vi "Random choice.vi"(11 "Selection Made":bool) -> (0 "Number Choice":dbl, 1 "shuffled names":string[](array[string]), 3 "Choice":string)   [LabVIEW 2018]
uses:
  d6d7d0bd-268b-43ab-82c5-82dfef68d144.vi
  <vilib>/Utility/file.llb/Read Delimited Spreadsheet (string).vi
  <vilib>/Utility/file.llb/Write Delimited Spreadsheet (string).vi
panel:
  out "Names":string[](array[string])
  out "number (0 to 1)":dbl
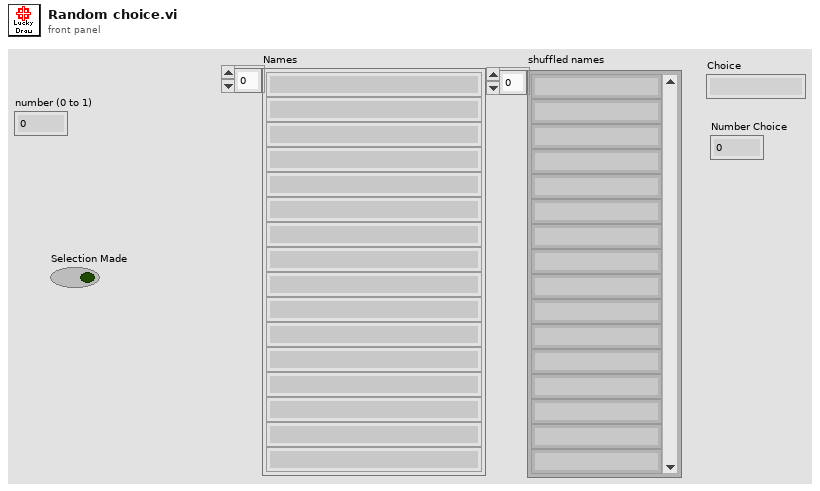
[diagram p1: front panel]
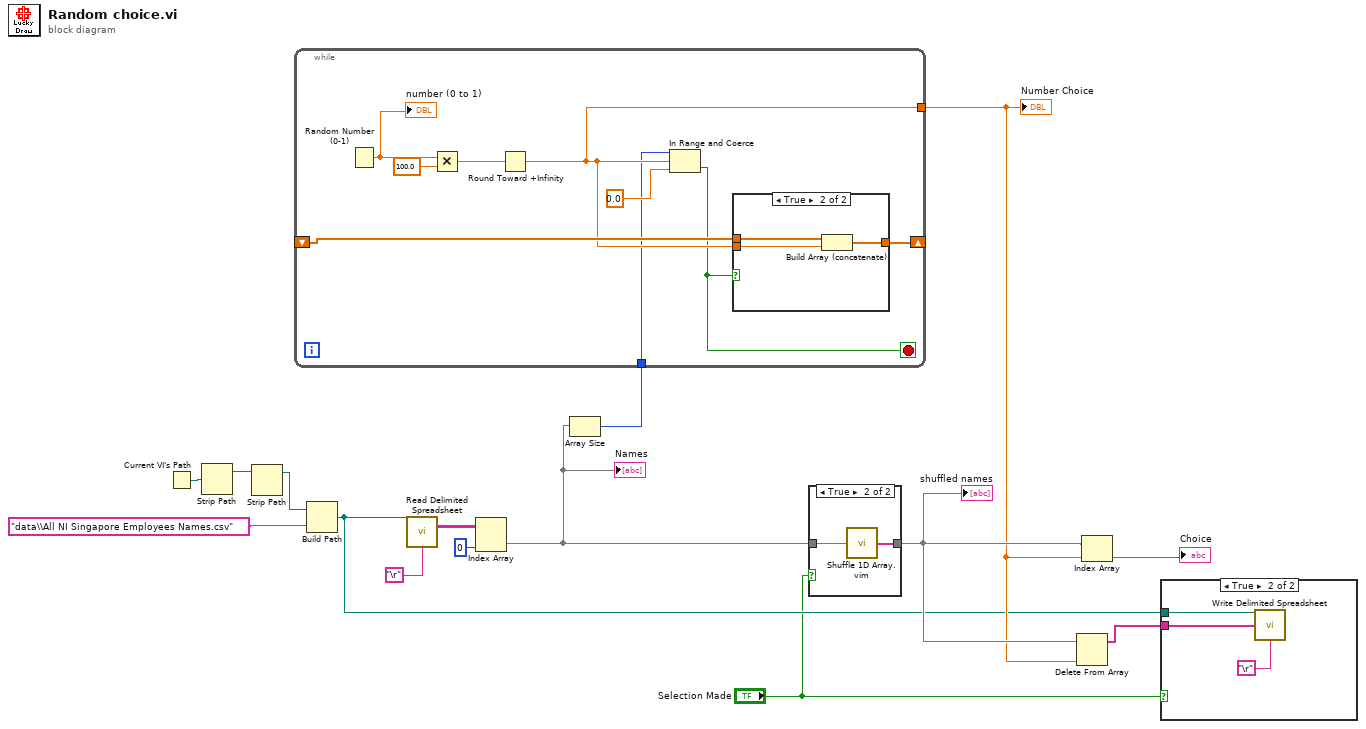
[diagram p0: block diagram]
diagram:
  n1 = Current VI's Path() -> (path=w15:path)
  n2 = Strip Path(path=w15) -> (stripped path=w14:path)  [unwired: 1 out]
  n3 = Strip Path(path=w14) -> (stripped path=w13:path)  [unwired: 1 out]
  n4 = Build Path(base path=w13, name or relative path="data\\All NI Singapore Employees Names.csv") -> (appended path=w5:path)
  n5 = call-poly <vilib>:"Read Delimited Spreadsheet.vi"("file path (dialog if empty)"=w5, "delimiter (\\t)"="\r") -> ("all rows"=w10:string[][])  [unwired: 8 in, 5 out]
  n6 = Index Array(array=w10, index (col)=0 ("disabled index (col)")) -> (element=w3:string[])  [unwired: 1 in]
  "Names" <- w3
  n7 = Array Size(array=w3) -> (size(s)=w2:i32)
  n8 = while {
    tunnel: [w18] -> w6
    shift-right: [w20] -> _
    shift-left: _ -> [w19]
    tunnel: w2 -> [w16]
    stop <- w17 stop-if-true
    n9 = Random Number (0-1)() -> (number: 0 to 1=w24:dbl)
    "number (0 to 1)" <- w24
    n10 = Multiply(x=w24, y=100.0) -> (x*y=w22:dbl)
    n11 = Round Toward +Infinity(x=w22) -> (ceil(x): smallest int >= x=w18:dbl)
    n12 = In Range and Coerce(upper limit=w16, x=w18, lower limit=0.0) -> (In Range?=w17:bool)  [unwired: 1 out]
    n13 = case shown="True" w17 {
      tunnel: [w25 w28] -> w20
      tunnel: w19 -> [w25 w27]
      tunnel: w18 -> [_ w26]
      frame False {
      }
      frame True {
        n14 = Build Array (concatenate)(w27, w26) -> (w28:dbl[])
      }
    }
  }
  "Number Choice" <- w6
  n15 = case shown="True" "Selection Made" {
    tunnel: [w29 w31] -> w7
    tunnel: w3 -> [w29 w30]
    frame False {
    }
    frame True {
      n16 = call "Shuffle 1D Array.vim"("array"=w30) -> ("shuffled array"=w31:string[])  [unwired: 4 in]
    }
  }
  "shuffled names" <- w7
  n17 = Delete From Array(array=w7, index=w6) -> (array with subset deleted=w4:string[])  [unwired: 1 in, 1 out]
  n18 = Index Array(array=w7, index=w6) -> (element=→"Choice":string)
  n19 = case shown="True" "Selection Made" {
    tunnel: w5 -> [_ w33]
    tunnel: w4 -> [_ w32]
    frame False {
    }
    frame True {
      n20 = call-poly <vilib>:"Write Delimited Spreadsheet.vi"("file path (dialog if empty)"=w33, "1D data"=w32, "delimiter (\\t)"="\r") -> ()  [unwired: 11 in, 2 out]
    }
  }
